vi "AFG3352X.remove services 2nd channel.vi"(0 "i ref in":refnum<vi>, 3 "ms timeout (10000)":i32=10000, 5 "error in (no error)":errorcluster) -> (14 "i ref out":refnum<vi>, 17 "timed out":bool, 19 "error out":errorcluster)   [LabVIEW 2014, in "AFG3352X.lvlib"]
doc: "Removes my DIM services."
uses:
  AFG3352X.lvlib
  CSlibraries-extern/DimLVEvent/LVDimInterface/LVDimInterface.lvlib
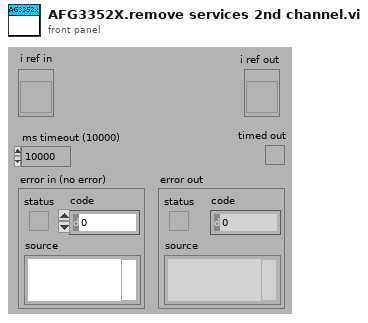
[diagram p1: front panel]
types:
  T1 = typedef "AFG3352X.lvlib/AFG3352X.i attribute.ctl" = cluster{"Act2ndValues":cluster{"frequency":dbl, "amplitude":dbl, "phase":dbl, "DCOffset":dbl, "waveformType":T2, "enableOutput":bool, "trigger":i16[], "serviceIDs":cluster{"frequencyID":i32, "amplitudeID":i32, "phaseID":i32, "DCOffsetID":i32, "waveformTypeID":i32, "enableOutputID":i32, "triggerID":i32}, "waveform":cluster{"data":waveform(dbl), "gain":dbl, "offset":dbl, "repetitionRate":dbl, "sampleRate":dbl}}, "Nom2ndValues":cluster{"frequency":dbl, "amplitude":dbl, "phase":dbl, "DCOffset":dbl, "waveformType":T2, "enableOutput":bool, "trigger":i16[], "serviceIDs":cluster{"frequencyID":i32, "amplitudeID":i32, "phaseID":i32, "DCOffsetID":i32, "waveformTypeID":i32, "enableOutputID":i32, "triggerID":i32}, "waveform":cluster{"data":waveform(dbl), "gain":dbl, "offset":dbl, "repetitionRate":dbl, "sampleRate":dbl}}, "DefaultChannel":i32, "ActAddValues":cluster{"Mode1":u16, "serviceIDs":cluster{"Mode1ID":i32, "Mode2ID":i32, "Burst1ID":i32, "Burst2ID":i32}, "Mode2":u16, "Burst1":i32, "Burst2":i32}, "NomAddValues":cluster{"Mode1":u16, "serviceIDs":cluster{"Mode1ID":i32, "Mode2ID":i32, "Burst1ID":i32, "Burst2ID":i32}, "Mode2 2":u16, "Burst1":i32, "Burst2":i32}, "enableBurstMode":bool}
  T2 = typedef "AFGBase.lvlib/AFGBase.waveformType.ctl" = enum16{"sine", "square", "ramp", "pulse", "noise", "DC", "arbitrary", "triangle", "ramp_up", "ramp_down", "amplitude modulation"}
  T3 = cluster{"frequencyID":i32, "amplitudeID":i32, "phaseID":i32, "DCOffsetID":i32, "waveformTypeID":i32, "enableOutputID":i32, "triggerID":i32}
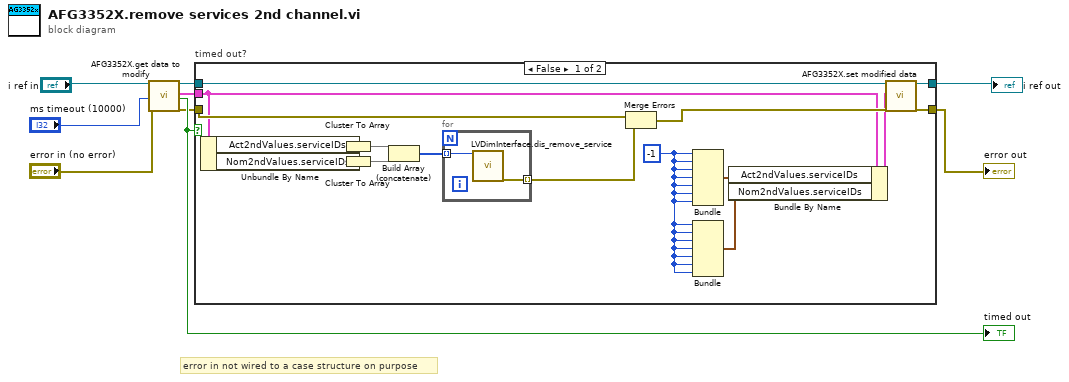
[diagram p0: block diagram]
diagram:
  # "error in not wired to a case structure on purpose"
  n1 = call "AFG3352X.get data to modify.vi"("i ref in"="i ref in", "ms timeout (10000)"="ms timeout (10000)", "error in (no error)"="error in (no error)") -> ("i ref out"=w5:refnum<vi>, "i attribute"=w3:T1, "timed out"=w6:bool, "error out"=w4:errorcluster)  [unwired: 13 in]
  "timed out" <- w6
  n2 = case "timed out?" shown="False" w6 {
    tunnel: w5 -> [w20 w29]
    tunnel: [w25 w29] -> w1
    tunnel: w4 -> [w23 w28]
    tunnel: [w24 w28] -> w8
    tunnel: w3 -> [w19 _]
    frame False {
      w11 = -1
      n3 = Unbundle By Name(w19) -> ("Act2ndValues.serviceIDs"=w18:T3, "Nom2ndValues.serviceIDs"=w17:T3)
      n4 = Cluster To Array(cluster=w18) -> (array=w16:i32[])
      n5 = Cluster To Array(cluster=w17) -> (array=w15:i32[])
      n6 = Build Array (concatenate)(w16, w15) -> (w13:i32[])
      n7 = for {
        tunnel: w13 -> [w27] mode=indexing
        tunnel: [w26] -> w12 mode=indexing
        n8 = call "LVDimInterface.dis_remove_service.vi"("my_serviceID"=w27) -> ("error out"=w26:errorcluster)  [unwired: 18 in]
      }
      n9 = Merge Errors(w23, w12) -> (w22:errorcluster)
      n10 = Bundle(w11, w11, w11, w11, w11, w11, w11) -> (w14:cluster{i32, i32, i32, i32, i32, i32, i32})  [unwired: 1 in]
      n11 = Bundle(w11, w11, w11, w11, w11, w11, w11) -> (w10:cluster{i32, i32, i32, i32, i32, i32, i32})  [unwired: 1 in]
      n12 = Bundle By Name(cluster=w19, "Act2ndValues.serviceIDs"=w14, "Nom2ndValues.serviceIDs"=w10) -> (w21:T1)
      n13 = call "AFG3352X.set modified data.vi"("i ref in"=w20, "i attribute"=w21, "error in (no error)"=w22) -> ("i ref out"=w25:refnum<vi>, "error out"=w24:errorcluster)  [unwired: 15 in]
    }
    frame True {
    }
  }
  "error out" <- w8
  "i ref out" <- w1
